vi "Write Section Data.vi"(6 "Insert If Not Exist(T)":bool=TRUE, 7 "Section Name":string, 8 "error in (no error)":errorcluster, 10 "Section Data":string[][](array[string]), 11 "Config Data":T1(array[cluster])=[{"Section Name"="General", "Section Data"=[["MatchSeqFile", "Hi6825RLIV100D.seq"], ["CorrOffsetFilePath", ""]]}, {"Section Name"="PluginCfg", "Section Data"=[]}, {"Section Name"="CompCfg", "Section Data"=[["Index", "TestName", "TestNumber", "NormVal", "Units", "Checked", "LowLimit", "HighLimit", "KUG_1"], ["1", "RF_Gain_ChA_HG_35001", "3", "0", "dBm", "T", "0", "0", "0"], ["2", "RF_Gain_ChB_HG_3500", "4", "0", "dBm", "T", "0", "0", "0"], ["3", "RF_NF_ChA_LG_3500", "5", "0", "", "T", "0", "0", "0"], ["4", "RF_NF_ChB_LG_3500", "6", "0", "", "T", "0", "0", "0"], ["5", "RF_NF_ChA_HG_3500", "7", "0", "", "T", "0", "0", "0"], ["6", "RF_NF_ChB_HG_3500", "8", "0", "", "T", "0", "0", "0"], ["7", "RF_InsertionLoss_ChA_3500", "9", "0", "dBm", "T", "0", "0", "0"], ["8", "RF_InsertionLoss_ChB_3500", "10", "0", "dBm", "T", "0", "0", "0"], ["9", "RF_InsertionLoss_CHA_FixedFreq_100", "11", "0", "dBm", "T", "0", "0", "0"], ["10", "RF_InsertionLoss_CHB_FixedFreq_100", "12", "0", "dBm", "T", "0", "0", "0"], ["11", "RF_Gain_ChA_HG_3500", "113", "0", "dBm", "T", "0", "0", "0"], ["12", "RF_Gain_ChB_HG_3500", "114", "0", "dBm", "T", "0", "0", "0"], ["13", "RF_NF_ChA_LG_3500", "115", "0", "", "T", "0", "0", "0"], ["14", "RF_NF_ChB_LG_3500", "116", "0", "", "T", "0", "0", "0"], ["15", "RF_NF_ChA_HG_3500", "117", "0", "", "T", "0", "0", "0"], ["16", "RF_NF_ChB_HG_3500", "118", "0", "", "T", "0", "0", "0"], ["17", "RF_InsertionLoss_ChA_3500", "119", "0", "dBm", "T", "0", "0", "0"], ["18", "RF_InsertionLoss_ChB_3500", "120", "0", "dBm", "T", "0", "0", "0"], ["19", "RF_InsertionLoss_CHA_FixedFreq_100", "121", "0", "dBm", "T", "0", "0", "0"], ["20", "RF_InsertionLoss_CHB_FixedFreq_100", "122", "0", "dBm", "T", "0", "0", "0"]]}]) -> (0 "error out":errorcluster, 3 "Config Data out":T1(array[cluster]))   [LabVIEW 2020, in "GUCalibration2.lvlib"]
uses:
  GUCalibration2.lvlib
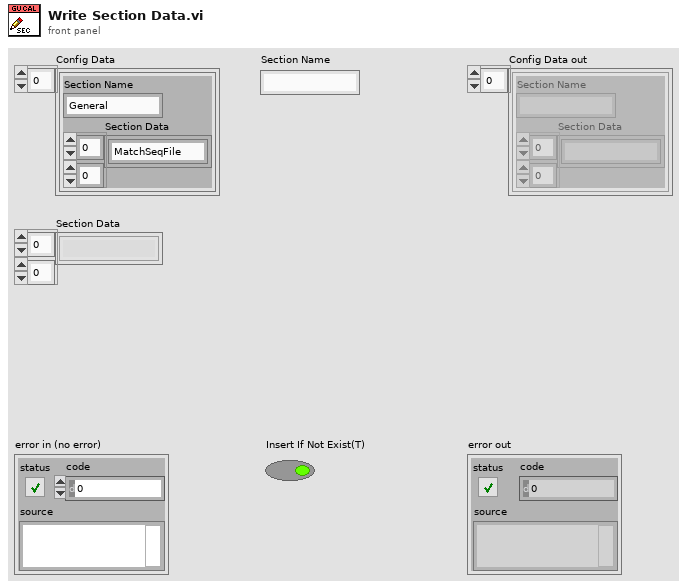
[diagram p1: front panel]
types:
  T1 = cluster{"Section Name":string, "Section Data":string[][]}[]
  T2 = cluster{"Section Name":string, "Section Data":string[][]}
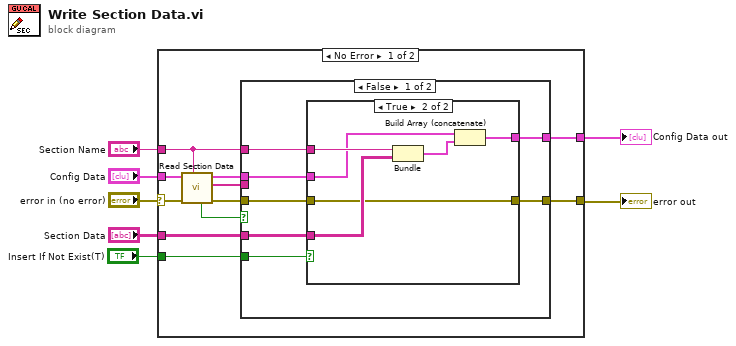
[diagram p0: block diagram]
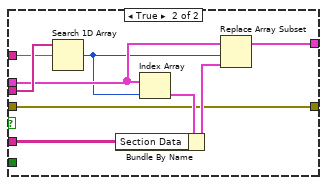
[diagram p3: hidden frame]
diagram:
  n1 = case shown="No Error" "error in (no error)" {
    selector: "error in (no error)" -> [w18 w44]
    tunnel: "Section Name" -> [w12 _]
    tunnel: "Config Data" -> [w17 w43]
    tunnel: [w9 w44] -> w4
    tunnel: [w10 w43] -> w3
    tunnel: "Section Data" -> [w11 _]
    tunnel: "Insert If Not Exist(T)" -> [w8 _]
    frame No Error {
      n2 = call "Read Section Data.vi"("Section Name"=w12, "error in (no error)"=w18, "Config Data"=w17) -> ("error out"=w15:errorcluster, "Section Names"=w13:string[], "Config Data out"=w14:T1, "Section Exist"=w16:bool)  [unwired: 4 in, 1 out]
      n3 = case shown="False" w16 {
        tunnel: w15 -> [w19 w34]
        tunnel: w14 -> [w23 w38]
        tunnel: w13 -> [_ w42]
        tunnel: w12 -> [w25 w41]
        tunnel: w11 -> [w24 w39]
        tunnel: [w22 w35] -> w10
        tunnel: [w20 w34] -> w9
        tunnel: w8 -> [w21 _]
        frame False {
          n4 = case shown="True" w21 {
            tunnel: w25 -> [_ w33]
            tunnel: w24 -> [_ w32]
            tunnel: w23 -> [w26 w31]
            tunnel: [w26 w29] -> w22
            tunnel: [w27 w28] -> w20
            tunnel: w19 -> [w27 w28]
            frame False {
            }
            frame True {
              n5 = Bundle("Section Name"=w33, "Section Data"=w32) -> (w30:T2)  [unwired: 1 in]
              n6 = Build Array (concatenate)(w31, w30) -> (w29:T1)
            }
          }
        }
        frame True {
          n7 = Search 1D Array(1D array=w42, element=w41) -> (index of element=w36:i32)  [unwired: 1 in]
          n8 = Index Array(array=w38, index=w36) -> (element=w40:T2)
          n9 = Bundle By Name(cluster=w40, "Section Data"=w39) -> (w37:T2)
          n10 = Replace Array Subset(array=w38, new element=w37, index=w36) -> (w35:T1)
        }
      }
    }
    frame Error {
    }
  }
  "error out" <- w4
  "Config Data out" <- w3
